vi "Read Waveform Measurement.vi"   [LabVIEW 2021, in "Siglent SDS 1000 2000 Series.lvlib"]
doc: "This VI selects the type of read: Standard or Px."
uses:
  <instrlib>/Siglent SDS 1000 2000 Series/Siglent SDS 1000 2000 Series.lvlib
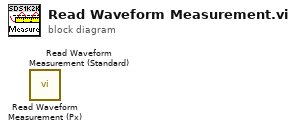
[diagram p0: block diagram]
diagram:
  n1 = call <instrlib>:"Read Waveform Measurement (Px).vi"() -> ()  [unwired: 13 in, 3 out]
  n2 = call <instrlib>:"Read Waveform Measurement (Standard).vi"() -> ()  [unwired: 13 in, 3 out]
